vi "parseReadBoosterValveGainError.vi"(8 "error in (no error)":errorcluster, 10 "DynamicFrameParser":refnum<class "DynamicFrameParser.lvclass">, 11 "FAILC in":refnum<class "FAILC.lvclass">) -> (0 "error out":errorcluster, 3 "FAILC out":refnum<class "FAILC.lvclass">)   [LabVIEW 2016, in "RTFAILC.lvlib" / "FAILC.lvclass"]
uses:
  FAILC.lvclass
  Common_RT_Modbus/DynamicFrameParser/DynamicFrameParser.lvclass
  FAILC.lvclass/FAILC.ctl
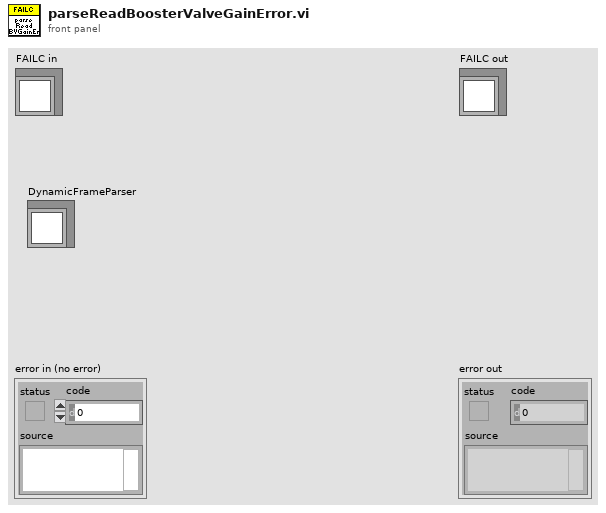
[diagram p1: front panel]
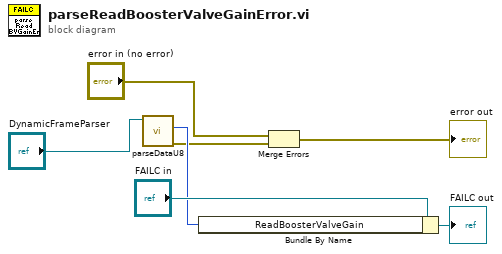
[diagram p0: block diagram]
diagram:
  n1 = call "parseDataU8.vi"("FrameParser in"="DynamicFrameParser") -> ("error out"=w4:errorcluster, "Data"=w5:u8)  [unwired: 8 in, 1 out]
  n2 = Bundle By Name(cluster="FAILC in", "ReadBoosterValveGain"=w5) -> (→"FAILC out":refnum<class "FAILC.lvclass">)
  n3 = Merge Errors("error in (no error)", w4) -> (→"error out":errorcluster)
